vi "Get Mux Config.vi"(8 "error in (no error)":errorcluster, 11 "Mux in":refnum<class "Mux.lvclass">) -> (0 "error out":errorcluster, 2 "Mux Config":T1, 3 "Mux out":refnum<class "Mux.lvclass">)   [LabVIEW 2022 SP3]
uses:
  Mux Config.ctl
  Mux.lvclass
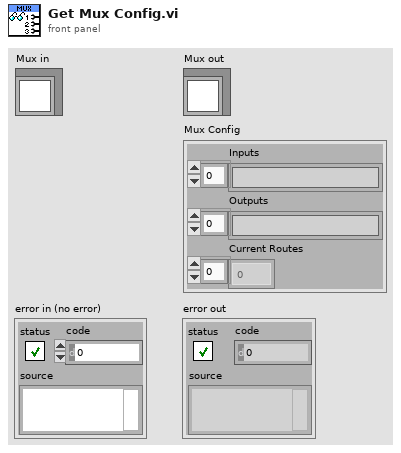
[diagram p1: front panel]
types:
  T1 = typedef "VideoMux.lvlib/Mux.lvclass/Mux Config.ctl" = cluster{"Inputs":string[], "Outputs":string[], "Current Routes":i32[]}
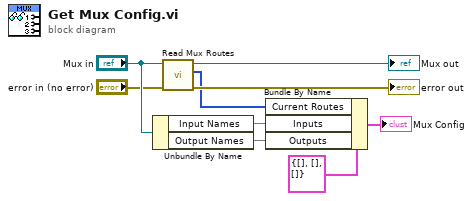
[diagram p0: block diagram]
diagram:
  n1 = Unbundle By Name("Mux in") -> ("Input Names"=w7, "Output Names"=w6)
  n2 = call-dynamic "Read Mux Routes.vi"("error in (no error)"="error in (no error)", "Mux in"="Mux in") -> ("error out"=→"error out":errorcluster, "Current Routes"=w1:i32[], "Mux out"=→"Mux out":refnum<class "Mux.lvclass">)  [unwired: 7 in]
  n3 = Bundle By Name(cluster=T1 {"Inputs"=[], "Outputs"=[], "Current Routes"=[]} ("System Config"), "Current Routes"=w1, "Inputs"=w7, "Outputs"=w6) -> (→"Mux Config":T1)
